vi "DeleteContained.vi"(8 "error in (no error)":errorcluster, 9 "Item to contain":refnum<class "ILabVIEWItem.lvclass">, 11 "CLabVIEWContainer in":refnum<class "CLabVIEWContainer.lvclass">) -> (0 "error out":errorcluster, 3 "CLabVIEWContainer out":refnum<class "CLabVIEWContainer.lvclass">)   [LabVIEW 2020, in "LabVIEWContainers.lvlib" / "CLabVIEWContainer.lvclass"]
uses:
  CLabVIEWContainer.lvclass
  CLabVIEWContainer.lvclass/CLabVIEWContainer.ctl
  LabVIEWObjectInterfaces/ILabVIEWItem/ILabVIEWItem.lvclass
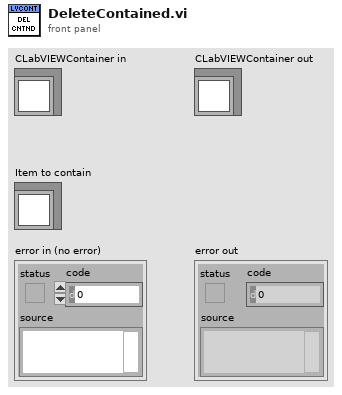
[diagram p1: front panel]
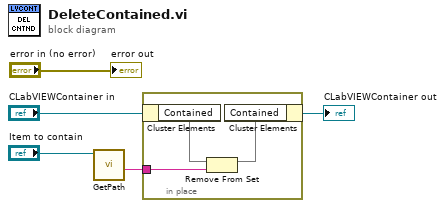
[diagram p0: block diagram]
diagram:
  n1 = call-dynamic "GetPath.vi"("ILabVIEWItem in"="Item to contain") -> ("Path"=w4:string)  [unwired: 8 in, 2 out]
  n2 = in-place {
    in-place-border: w4 -> [w6]
    n3 = in-place-cluster #1("CLabVIEWContainer in") -> ("Contained"=w7:set{string})
    n4 = Remove From Set(10:w6, 11:w7) -> (3:w8:set{string})  [unwired: 1 out]
    n5 = in-place-cluster #1("Contained"=w8) -> (→"CLabVIEWContainer out":refnum<class "CLabVIEWContainer.lvclass">)
  }
  "error out" <- "error in (no error)"
